vi "Comm Disconnect.vi"(8 "error in (no error)":errorcluster, 11 "niDTS Comm Serial in":refnum<class "niDTS Comm Serial.lvclass">) -> (0 "error out":errorcluster, 3 "niDTS Comm Serial out":refnum<class "niDTS Comm Serial.lvclass">)   [LabVIEW 2015, in "niDTS CommLib.lvlib" / "niDTS Comm Serial.lvclass"]
uses:
  niDTS Comm Serial.lvclass
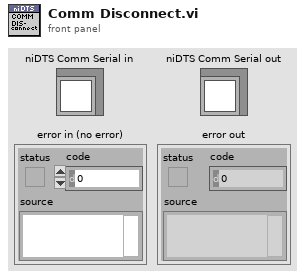
[diagram p1: front panel]
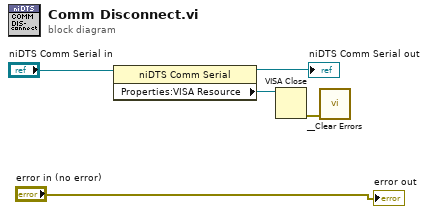
[diagram p0: block diagram]
diagram:
  n1 = property class="niDTS Comm Serial"(reference="niDTS Comm Serial in") -> (reference out=→"niDTS Comm Serial out":refnum<class "niDTS Comm Serial.lvclass">, "Properties:VISA Resource"=w3:refnum<visa-resource-name>)  [unwired: 1 in, 1 out]
  n2 = VISA Close(VISA resource name=w3) -> (error out=w1:errorcluster)  [unwired: 1 in]
  n3 = call "__Clear Errors.vi"("error in (no error)"=w1) -> ()  [unwired: 5 in, 2 out]
  "error out" <- "error in (no error)"
